vi "rad_Reboot (IP) Wrapper.vi"(8 "error in (no error)":errorcluster, 10 "wait for restart? (F)":bool, 11 "Target settings in":T1={"Hostname"="", "Serial number"="", "Product name"="", "Product code"=0, "System status"="", "Credential type"=enum."None/Unlocked", "User added?"=FALSE, "Primary NIC"={"MAC address"="", "IP Address Request Mode"=2, "IP address"="", "Subnet mask"="", "Gateway"="", "DNS server"=""}} {"Primary NIC"."IP Address Request Mode" items=["Static"=1, "DHCP/Link-Local"=2, "Link-Local Only"=4, "DHCP Only"=8]}) -> (0 "error out":errorcluster, 3 "Target settings out":T1={"Hostname"="", "Serial number"="", "Product name"="", "Product code"=0, "System status"="", "Credential type"=enum."None/Unlocked", "User added?"=FALSE, "Primary NIC"={"MAC address"="", "IP Address Request Mode"=2, "IP address"="", "Subnet mask"="", "Gateway"="", "DNS server"=""}} {"Primary NIC"."IP Address Request Mode" items=["Static"=1, "DHCP/Link-Local"=2, "Link-Local Only"=4, "DHCP Only"=8]})   [LabVIEW 2020]
uses:
  Targets/TypeDefs/rad_Target Information.ctl
  Targets/TypeDefs/rad_Target Network Settings.ctl
  <vilib>/nisyscfg/Close (System).vi
  <vilib>/nisyscfg/nisyscfg.lvlib
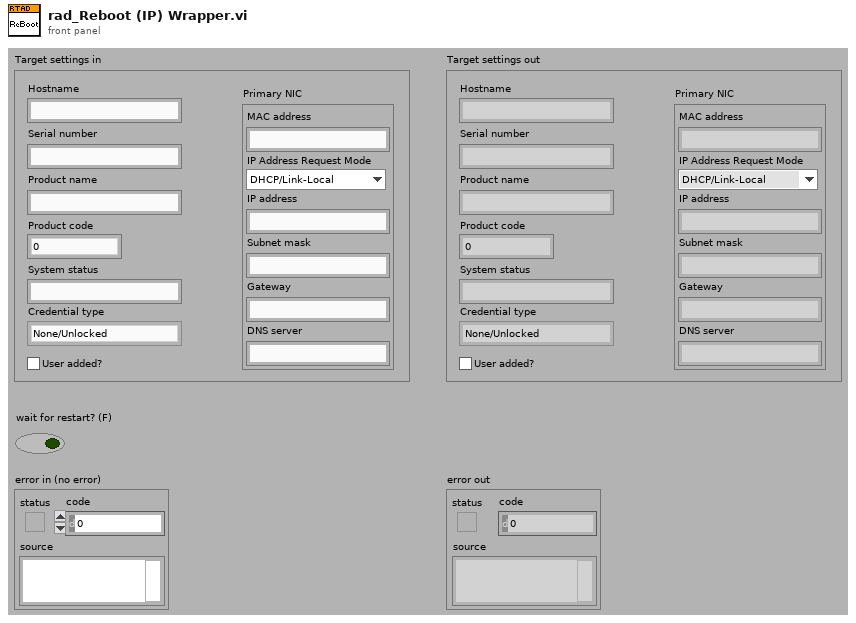
[diagram p1: front panel]
types:
  T1 = typedef "rad_Target Information.ctl" = cluster{"Hostname":string, "Serial number":string, "Product name":string, "Product code":i32, "System status":string, "Credential type":enum16{"None/Unlocked", "FTP Password", "NIAuth Credentials"}, "User added?":bool, "Primary NIC":T2}
  T2 = typedef "rad_Target Network Settings.ctl" = cluster{"MAC address":string, "IP Address Request Mode":i32, "IP address":string, "Subnet mask":string, "Gateway":string, "DNS server":string}
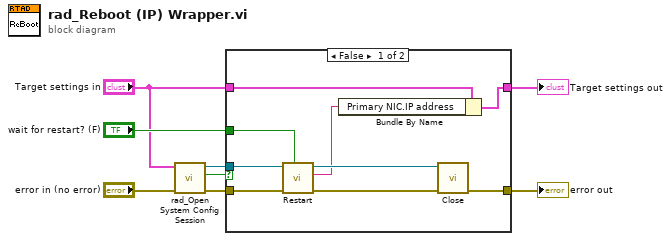
[diagram p0: block diagram]
diagram:
  n1 = call "rad_Open System Config Session.vi"("error in (no error)"="error in (no error)", "Target settings"="Target settings in") -> ("error out"=w3:errorcluster, "Cancelled"=w5:bool, "Session out"=w4:refnum<k21>)  [unwired: 6 in, 1 out]
  n2 = case shown="False" w5 {
    tunnel: "wait for restart? (F)" -> [w17 _]
    tunnel: [w12 w19] -> w6
    tunnel: w4 -> [w16 _]
    tunnel: w3 -> [w15 w19]
    tunnel: "Target settings in" -> [w11 w18]
    tunnel: [w10 w18] -> w1
    frame False {
      n3 = call <vilib>:"Restart.vi"("Wait Until Complete (T)"=w17, "error in (no error)"=w15, "Session in"=w16) -> ("error out"=w13:errorcluster, "New IP Address"=w9:string, "Session out"=w14:refnum<k21>)  [unwired: 6 in]
      n4 = Bundle By Name(cluster=w11, "Primary NIC.IP address"=w9) -> (w10:T1)
      n5 = call-poly <vilib>:"Close.vi"("error in (no error)"=w13, "Session in"=w14) -> ("error out"=w12:errorcluster)  [unwired: 9 in]
    }
    frame True {
    }
  }
  "error out" <- w6
  "Target settings out" <- w1
